vi "PH_BeamlineInformation.set GUI Refs.vi"(0 "Ref in":refnum<vi>, 1 "Class":string, 2 "BeamlineInformation GUI Refs":T1={"BL Elements"=[], "Powermeters"={"ns FE"={"GUI Ref"=refnum, "Value"=-1.0}, "fs FE"={"GUI Ref"=refnum, "Value"=-1.0}, "PA"={"GUI Ref"=refnum, "Value"=-1.0}, "MA"={"GUI Ref"=refnum, "Value"=-1.0}, "Z6 green"={"GUI Ref"=refnum, "Value"=-1.0}, "Z6 IR"={"GUI Ref"=refnum, "Value"=-1.0}, "Z6 COS"={"GUI Ref"=refnum, "Value"=-1.0}}, "Efficiency GUI Refs"={"PA Gain"={"GUI Ref"=refnum, "Value"=-1.0}, "MA Gain"={"GUI Ref"=refnum, "Value"=-1.0}, "Z6 green Conversion"={"GUI Ref"=refnum, "Value"=-1.0}, "Z6 Comp Losses"={"GUI Ref"=refnum, "Value"=-1.0}}, "Head GUI Refs"={"PA - 19 - 1"={"in Use"=refnum, "voltage"=refnum}, "PA - 19 - 2"={"in Use"=refnum, "voltage"=refnum}, "PA - 45"={"in Use"=refnum, "voltage"=refnum}, "PA - 45 - DP"={"in Use"=refnum, "voltage"=refnum}, "MA - 1"={"in Use"=refnum, "voltage"=refnum}, "MA - 2"={"in Use"=refnum, "voltage"=refnum}, "MA - 3"={"in Use"=refnum, "voltage"=refnum}, "MA - 4"={"in Use"=refnum, "voltage"=refnum}, "MA - 5"={"in Use"=refnum, "voltage"=refnum}, "MA - FR"={"in Use"=refnum, "voltage"=refnum}}, "System Information GUI Refs"={"Laser"=refnum, "PreAmp"=refnum, "MainAmp"=refnum, "Emergency Off"=refnum, "Exp 1"=refnum, "Exp 2"=refnum, "Exp 3"=refnum, "Exp 4"=refnum, "Timing Mode GUI Ref"=refnum}}, 5 "error in":errorcluster) -> (14 "Ref out":refnum<vi>, 19 "error out":errorcluster)   [LabVIEW 2014, in "PH_BeamlineInformation.lvlib"]
uses:
  PH_BeamlineInformation.lvlib
  PH_BeamlineInformation.GUI Ref.ctl
  PH_Beamline_Chief/PH_Beamline_Chief.Section.ctl
  PH_BeamlineInformation.Powermeter.ctl
  PH_BeamlineInformation.Efficiency.ctl
  PH_SystemInformation/PH_SystemInformation.GUI Refs.ctl
  PH_PP_Common/PH_PP_Common.PUs.ctl
  PH_BeamlineInformation.Head.ctl
  PH_Beamline_Chief/PH_Beamline_Chief.lvlib
  PH_PP_Common/PH_PP_Common.lvlib
  PH_SystemInformation/PH_SystemInformation.lvlib
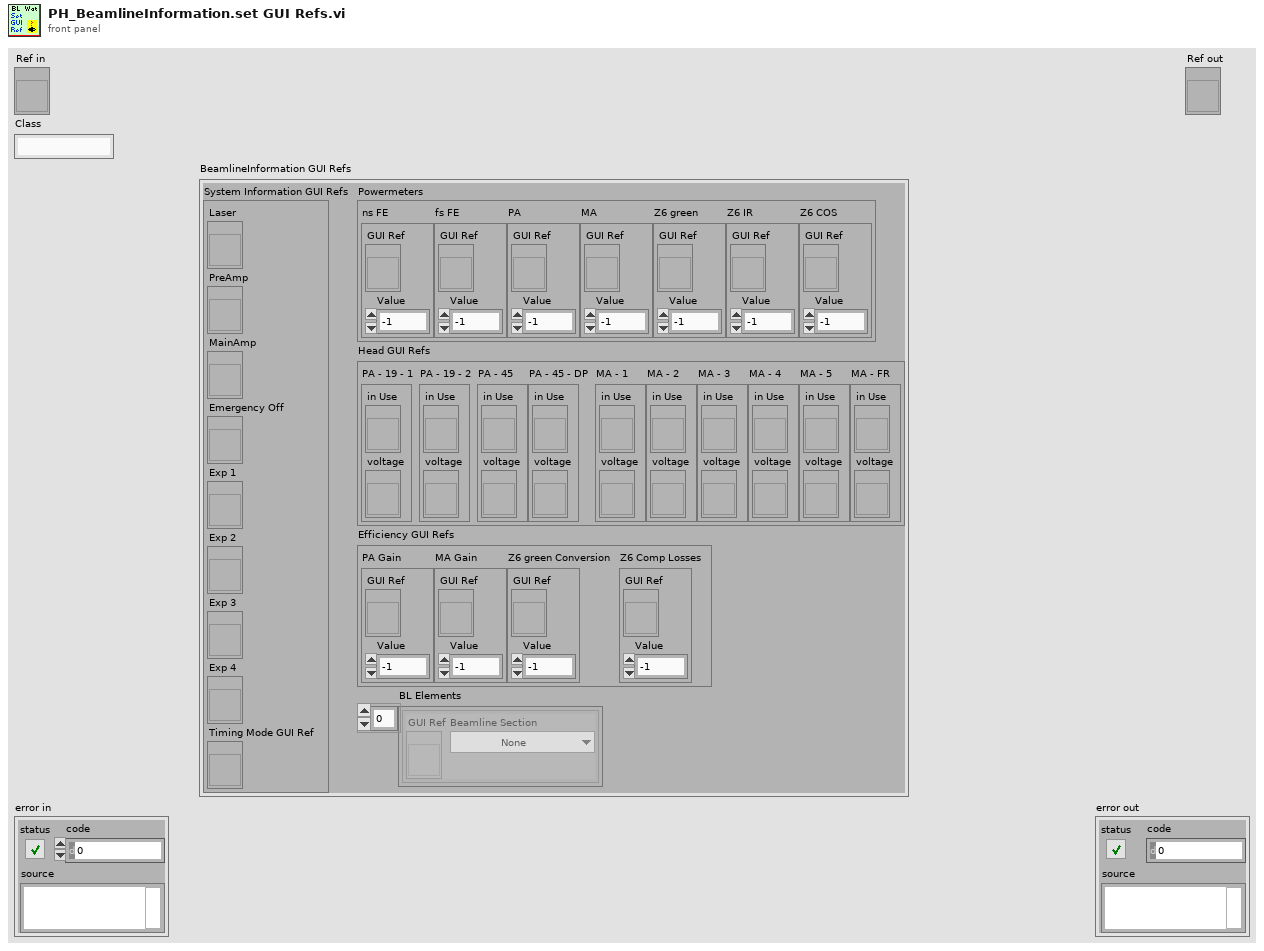
[diagram p1: front panel]
types:
  T1 = typedef "PH_BeamlineInformation.lvlib/PH_BeamlineInformation.GUI Ref.ctl" = cluster{"BL Elements":cluster{"GUI Ref":refnum<vi>, "Beamline Section":T2}[], "Powermeters":T3, "Efficiency GUI Refs":T4, "Head GUI Refs":cluster{"PA - 19 - 1":cluster{"in Use":refnum<vi>, "voltage":refnum<vi>}, "PA - 19 - 2":cluster{"in Use":refnum<vi>, "voltage":refnum<vi>}, "PA - 45":cluster{"in Use":refnum<vi>, "voltage":refnum<vi>}, "PA - 45 - DP":cluster{"in Use":refnum<vi>, "voltage":refnum<vi>}, "MA - 1":cluster{"in Use":refnum<vi>, "voltage":refnum<vi>}, "MA - 2":cluster{"in Use":refnum<vi>, "voltage":refnum<vi>}, "MA - 3":cluster{"in Use":refnum<vi>, "voltage":refnum<vi>}, "MA - 4":cluster{"in Use":refnum<vi>, "voltage":refnum<vi>}, "MA - 5":cluster{"in Use":refnum<vi>, "voltage":refnum<vi>}, "MA - FR":cluster{"in Use":refnum<vi>, "voltage":refnum<vi>}}, "System Information GUI Refs":T5}
  T2 = typedef "PH_Beamline_Chief.lvlib/PH_Beamline_Chief.Section.ctl" = enum16{"None", "YLF", "fs", "fs-YLF", "ns", "PA-Input", "PA-Undelay", "PA-Delay", "PA-before-Bypass", "PA", "PA-Bypass", "PA-Exit", "PA-LL", "LL", "PA-MA", "MA-Exit", "MA-Z6", "Z6", "MA-LB", "LB-TB2", "LB-TB3"}
  T3 = typedef "PH_BeamlineInformation.lvlib/PH_BeamlineInformation.Powermeter.ctl" = cluster{"ns FE":cluster{"GUI Ref":refnum<vi>, "Value":dbl}, "fs FE":cluster{"GUI Ref":refnum<vi>, "Value":dbl}, "PA":cluster{"GUI Ref":refnum<vi>, "Value":dbl}, "MA":cluster{"GUI Ref":refnum<vi>, "Value":dbl}, "Z6 green":cluster{"GUI Ref":refnum<vi>, "Value":dbl}, "Z6 IR":cluster{"GUI Ref":refnum<vi>, "Value":dbl}, "Z6 COS":cluster{"GUI Ref":refnum<vi>, "Value":dbl}}
  T4 = typedef "PH_BeamlineInformation.lvlib/PH_BeamlineInformation.Efficiency.ctl" = cluster{"PA Gain":cluster{"GUI Ref":refnum<vi>, "Value":dbl}, "MA Gain":cluster{"GUI Ref":refnum<vi>, "Value":dbl}, "Z6 green Conversion":cluster{"GUI Ref":refnum<vi>, "Value":dbl}, "Z6 Comp Losses":cluster{"GUI Ref":refnum<vi>, "Value":dbl}}
  T5 = typedef "PH_SystemInformation.lvlib/PH_SystemInformation.GUI Refs.ctl" = cluster{"Laser":refnum<vi>, "PreAmp":refnum<vi>, "MainAmp":refnum<vi>, "Emergency Off":refnum<vi>, "Exp 1":refnum<vi>, "Exp 2":refnum<vi>, "Exp 3":refnum<vi>, "Exp 4":refnum<vi>, "Timing Mode GUI Ref":refnum<vi>}
  T6 = typedef "PH_BeamlineInformation.lvlib/PH_BeamlineInformation.Head.ctl" = cluster{"PowerUnit":T7, "in use":cluster{"Value":bool, "GUI Ref":refnum<vi>, "linked":bool}, "voltage":cluster{"Value":dbl, "GUI Ref":refnum<vi>, "linked":bool}}
  T7 = typedef "PH_PP_Common.lvlib/PH_PP_Common.PUs.ctl" = enum16{"no Info", "PA-19mm-1", "PA-19mm-2", "PA-45mm-PILC", "PA-45mm-MAIN", "MA-PU-1", "MA-PU-2", "MA-PU-3", "MA-PU-4", "MA-PU-5", "MA-PU-6", "MA-FR", "MA-PILC", "PA-45mm-DP"}
  T8 = cluster{"Service Name":string, "GUI Elements":refnum<vi>[], "Status":i32}
  T9 = cluster{"PA - 19 - 1":cluster{"in Use":refnum<vi>, "voltage":refnum<vi>}, "PA - 19 - 2":cluster{"in Use":refnum<vi>, "voltage":refnum<vi>}, "PA - 45":cluster{"in Use":refnum<vi>, "voltage":refnum<vi>}, "PA - 45 - DP":cluster{"in Use":refnum<vi>, "voltage":refnum<vi>}, "MA - 1":cluster{"in Use":refnum<vi>, "voltage":refnum<vi>}, "MA - 2":cluster{"in Use":refnum<vi>, "voltage":refnum<vi>}, "MA - 3":cluster{"in Use":refnum<vi>, "voltage":refnum<vi>}, "MA - 4":cluster{"in Use":refnum<vi>, "voltage":refnum<vi>}, "MA - 5":cluster{"in Use":refnum<vi>, "voltage":refnum<vi>}, "MA - FR":cluster{"in Use":refnum<vi>, "voltage":refnum<vi>}}
  T10 = cluster{"GUI Ref":refnum<vi>, "Beamline Section":T2}[]
  T11 = cluster{"in Use":refnum<vi>, "voltage":refnum<vi>}[]
  T12 = typedef "PH_BeamlineInformation.lvlib/PH_BeamlineInformation.i attribute.ctl" = cluster{"BL GUI Elements of Services":cluster{"Service Name":string, "GUI Elements":refnum<vi>[], "Status":i32}[], "Powermeters":T3, "Efficiency":T4, "Heads":T6[]}
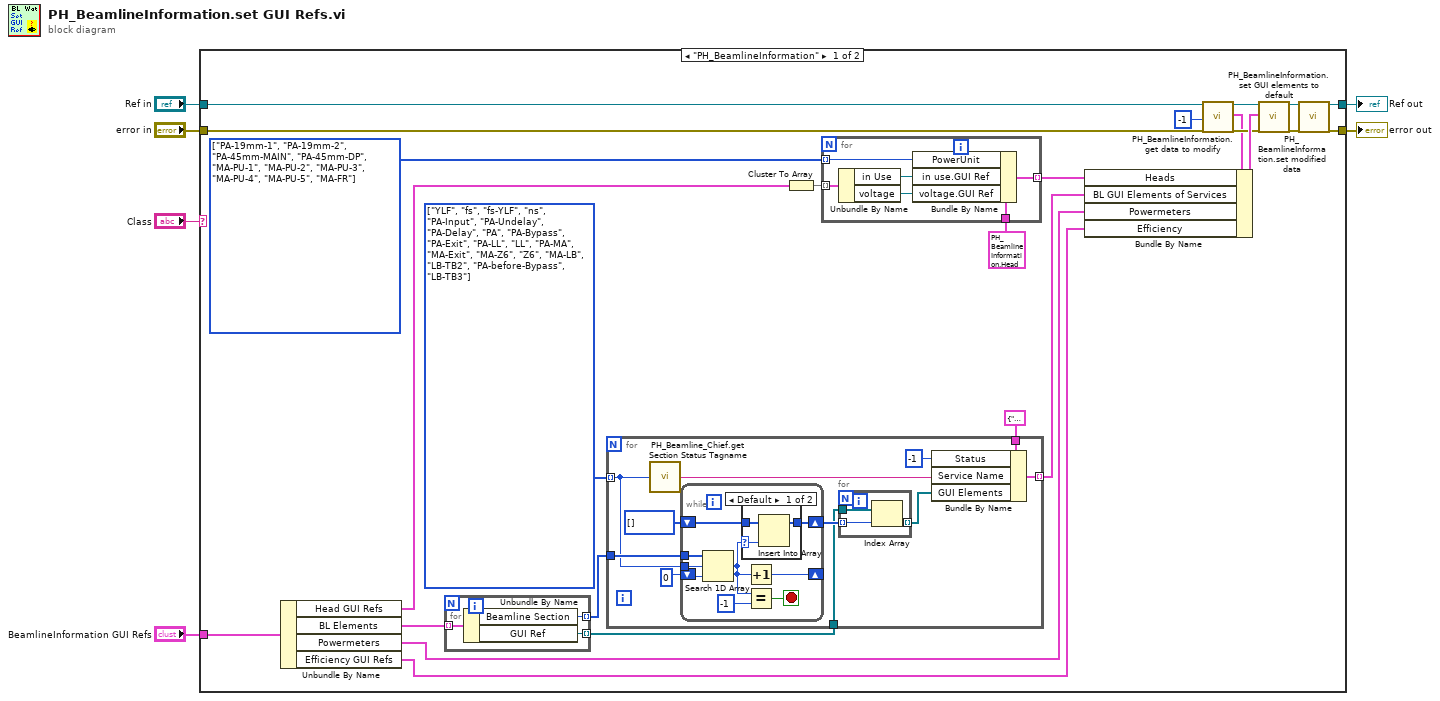
[diagram p0: block diagram]
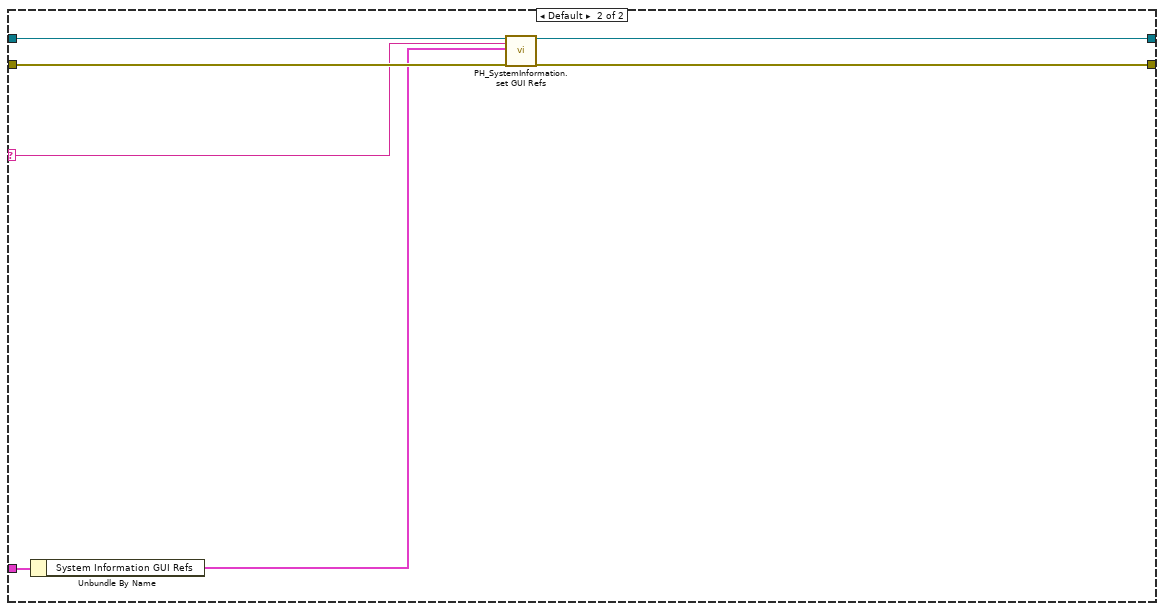
[diagram p3: hidden frame]
diagram:
  n1 = case shown="\"PH_BeamlineInformation\"" "Class" {
    selector: "Class" -> [_ w68]
    tunnel: "error in" -> [w30 w73]
    tunnel: "Ref in" -> [w29 w74]
    tunnel: [w8 w72] -> w4
    tunnel: [w7 w71] -> w3
    tunnel: "BeamlineInformation GUI Refs" -> [w15 w70]
    frame "PH_BeamlineInformation" {
      w18 = T7[] [enum."PA-19mm-1", enum."PA-19mm-2", enum."PA-45mm-MAIN", enum."PA-45mm-DP", enum."MA-PU-1", enum."MA-PU-2", enum."MA-PU-3", enum."MA-PU-4", enum."MA-PU-5", enum."MA-FR"] items=["no Info", "PA-19mm-1", "PA-19mm-2", "PA-45mm-PILC", "PA-45mm-MAIN", "MA-PU-1", "MA-PU-2", "MA-PU-3", "MA-PU-4", "MA-PU-5", "MA-PU-6", "MA-FR", "MA-PILC", "PA-45mm-DP"]
      w31 = T2[] [enum."YLF", enum."fs", enum."fs-YLF", enum."ns", enum."PA-Input", enum."PA-Undelay", enum."PA-Delay", enum."PA", enum."PA-Bypass", enum."PA-Exit", enum."PA-LL", enum."LL", enum."PA-MA", enum."MA-Exit", enum."MA-Z6", enum."Z6", enum."MA-LB", enum."LB-TB2", enum."PA-before-Bypass", enum."LB-TB3"] items=["None", "YLF", "fs", "fs-YLF", "ns", "PA-Input", "PA-Undelay", "PA-Delay", "PA-before-Bypass", "PA", "PA-Bypass", "PA-Exit", "PA-LL", "LL", "PA-MA", "MA-Exit", "MA-Z6", "Z6", "MA-LB", "LB-TB2", "LB-TB3"]
      n2 = Unbundle By Name(w15) -> ("Head GUI Refs"=w11:T9, "BL Elements"=w14:T10, "Powermeters"=w13:T3, "Efficiency GUI Refs"=w12:T4)
      n3 = for {
        tunnel: w14 -> [w40] mode=indexing
        tunnel: [w39] -> w22 mode=indexing
        tunnel: [w38] -> w21 mode=indexing
        n4 = Unbundle By Name(w40) -> ("Beamline Section"=w39:T2, "GUI Ref"=w38:refnum<vi>)
      }
      n5 = for {
        tunnel: [w51] -> w23 mode=indexing
        tunnel: T8 {"Service Name"="", "GUI Elements"=[], "Status"=0} ("Cluster") -> [w50]
        tunnel: w31 -> [w47] mode=indexing
        tunnel: w22 -> [w48]
        tunnel: w21 -> [w42]
        n6 = call "PH_Beamline_Chief.get Section Status Tagname.vi"("Beamline Section"=w47) -> ("Section Status Tagname"=w49:string)
        n7 = while {
          tunnel: w47 -> [w62]
          shift-right: [w61] -> w43
          shift-left: i32[] [] -> [w60]
          tunnel: w48 -> [w63]
          shift-right: [w58] -> _
          shift-left: 0 -> [w59]
          stop <- w55 stop-if-true
          n8 = Search 1D Array(1D array=w63, element=w62, start index (0)=w59) -> (index of element=w57:i32)
          n9 = case shown="Default" w57 {
            selector: w57 -> [w64 _]
            tunnel: [w66 w67] -> w61
            tunnel: w60 -> [w65 w67]
            frame Default {
              n10 = Insert Into Array(array=w65, new element=w64) -> (w66:i32[])  [unwired: 1 in]
            }
            frame -1 {
            }
          }
          n11 = Increment(x=w57) -> (x+1=w58:i32)
          n12 = Equal?(x=w57, y=-1) -> (x = y?=w55:bool)
        }
        n13 = for {
          tunnel: w43 -> [w54] mode=indexing
          tunnel: w42 -> [w53]
          tunnel: [w52] -> w41 mode=indexing
          n14 = Index Array(array=w53, index=w54) -> (element=w52:refnum<vi>)
        }
        n15 = Bundle By Name(cluster=w50, "Status"=-1, "Service Name"=w49, "GUI Elements"=w41) -> (w51:T8)
      }
      n16 = Cluster To Array(cluster=w11) -> (array=w19:T11)
      n17 = for {
        tunnel: w19 -> [w37] mode=indexing
        tunnel: w18 -> [w33] mode=indexing
        tunnel: T6 {"PowerUnit"=enum."no Info", "in use"={"Value"=FALSE, "GUI Ref"=refnum, "linked"=FALSE}, "voltage"={"Value"=0.0, "GUI Ref"=refnum, "linked"=FALSE}} ("Head") -> [w34]
        tunnel: [w32] -> w16 mode=indexing
        n18 = Unbundle By Name(w37) -> ("in Use"=w36:refnum<vi>, "voltage"=w35:refnum<vi>)
        n19 = Bundle By Name(cluster=w34, "PowerUnit"=w33, "in use.GUI Ref"=w36, "voltage.GUI Ref"=w35) -> (w32:T6)
      }
      n20 = call "PH_BeamlineInformation.get data to modify.vi"("i ref in"=w29, "ms timeout (10000)"=-1, "error in (no error)"=w30) -> ("i ref out"=w27:refnum<vi>, "i attribute"=w20:T12, "error out"=w25:errorcluster)  [unwired: 13 in, 1 out]
      n21 = Bundle By Name(cluster=w20, "Heads"=w16, "BL GUI Elements of Services"=w23, "Powermeters"=w13, "Efficiency"=w12) -> (w28:T12)
      n22 = call "PH_BeamlineInformation.set modified data.vi"("i ref in"=w27, "i attribute"=w28, "error in (no error)"=w25) -> ("i ref out"=w10:refnum<vi>, "error out"=w9:errorcluster)  [unwired: 15 in]
      n23 = call "PH_BeamlineInformation.set GUI elements to default.vi"("i ref in"=w10, "error in (no error)"=w9) -> ("i ref out"=w8:refnum<vi>, "error out"=w7:errorcluster)  [unwired: 16 in]
    }
    frame Default {
      n24 = Unbundle By Name(w70) -> ("System Information GUI Refs"=w69:T5)
      n25 = call "PH_SystemInformation.set GUI Refs.vi"("i ref in"=w74, "Class"=w68, "System Information GUI Refs"=w69, "error in (no error)"=w73) -> ("i ref out"=w72:refnum<vi>, "error out"=w71:errorcluster)  [unwired: 14 in]
    }
  }
  "error out" <- w3
  "Ref out" <- w4
